vi "De Jitter Data.vi"(10 "Target Info":dbl[][](array[numeric]) format="%#.1f") -> (2 "Filtered Data":dbl[][](array[numeric]))   [LabVIEW 2025]
panel:
  # "Distance"
  # "Angle"
  # "Tag #"
  # "Yaw"
  # "Pitch"
  # "Roll"
  # "Camera #"
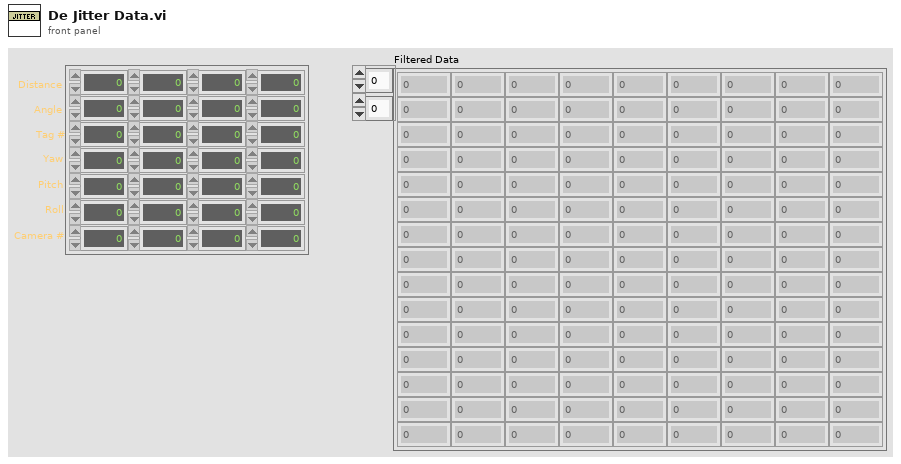
[diagram p1: front panel]
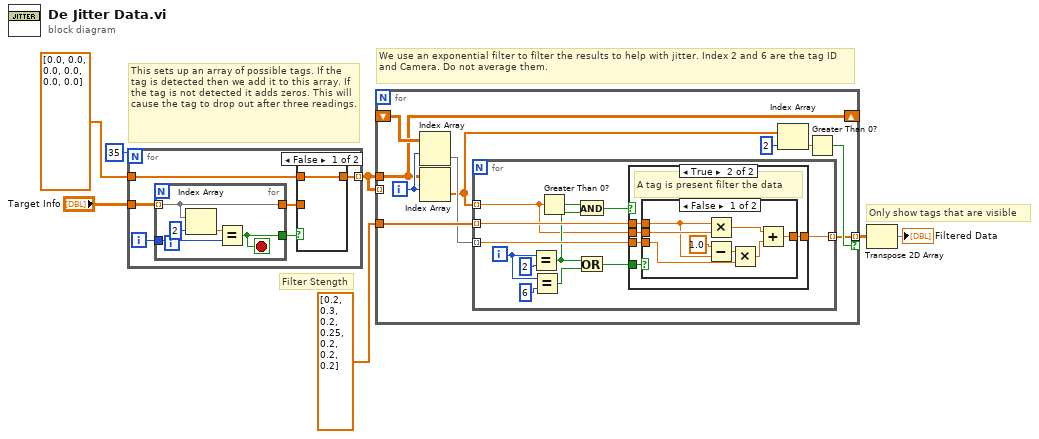
[diagram p0: block diagram]
diagram:
  # "Filter Stength"
  # "Only show tags that are visible"
  # "We use an exponential filter to filter the results to help with jitter. Index 2 and 6 are the tag ID and Camera. Do not average them."
  # "This sets up an array of possible tags. If the tag is detected then we add it to this array. If the tag is not detected it adds zeros. This will cause the tag to drop out after three readings."
  n1 = for {
    N: 35 -> [_]
    tunnel: dbl[] [0.0, 0.0, 0.0, 0.0, 0.0, 0.0] ("f") -> [w10]
    tunnel: "Target Info" -> [w11]
    tunnel: [w9] -> w3 mode=indexing
    i -> [w8]
    n2 = for {
      tunnel: [w15] -> w13
      tunnel: [w16] -> w12
      tunnel: w11 -> [w16] mode=indexing
      tunnel: w8 -> [w17]
      stop <- w15 stop-if-true
      n3 = Index Array(array=w16, index=2) -> (element=w18:dbl)
      n4 = Equal?(x=w18, y=w17) -> (x = y?=w15:bool)
    }
    n5 = case shown="False" w13 {
      tunnel: w12 -> [_ w20]
      tunnel: [w19 w20] -> w9
      tunnel: w10 -> [w19 _]
      frame False {
      }
      frame True {
      }
    }
  }
  n6 = for {
    tunnel: w3 -> [w21]
    shift-right: [w21] -> _
    shift-left: _ -> [w30]
    tunnel: [w28] -> w4 mode=indexing if=w29
    tunnel: w3 -> [_] mode=indexing
    tunnel: dbl[] [0.2, 0.3, 0.2, 0.25, 0.2, 0.2, 0.2] -> [w27]
    i -> [w26]
    n7 = Index Array(array=w30, index (row)=w26) -> (element=w23:dbl[])  [unwired: 1 in]
    n8 = Index Array(array=w21, index (row)=w26) -> (element=w22:dbl[])  [unwired: 1 in]
    n9 = for {
      tunnel: w22 -> [w31] mode=indexing
      tunnel: w23 -> [w42] mode=indexing
      tunnel: [w41] -> w28 mode=indexing
      tunnel: w27 -> [w36] mode=indexing
      i -> [w32]
      n10 = Equal?(x=w32, y=2) -> (x = y?=w34:bool)
      n11 = Equal?(x=w32, y=6) -> (x = y?=w38:bool)
      n12 = Greater Than 0?(x=w31) -> (x > 0?=w33:bool)
      n13 = And(x=w33, y=w34) -> (x .and. y?=w35:bool)
      n14 = Or(x=w34, y=w38) -> (x .or. y?=w37:bool)
      n15 = case shown="True" w35 {
        tunnel: w31 -> [_ w48]
        tunnel: w42 -> [w43 w47]
        tunnel: [w43 w46] -> w41
        tunnel: w37 -> [_ w45]
        tunnel: w36 -> [_ w44]
        frame False {
          # "Tag is 0 Use the previous data"
        }
        frame True {
          # "A tag is present filter the data"
          n16 = case shown="False" w45 {
            tunnel: w48 -> [w56 _]
            tunnel: w47 -> [w53 w57]
            tunnel: [w50 w57] -> w46
            tunnel: w44 -> [w49 _]
            frame False {
              n17 = Multiply(x=w49, y=w56) -> (x*y=w51:dbl)
              n18 = Subtract(x=1.0, y=w49) -> (x-y=w54:dbl)
              n19 = Multiply(x=w54, y=w53) -> (x*y=w52:dbl)
              n20 = Add(x=w51, y=w52) -> (x+y=w50:dbl)
            }
            frame True {
            }
          }
        }
      }
    }
    n21 = Index Array(array=w22, index=2) -> (element=w24:dbl)
    n22 = Greater Than 0?(x=w24) -> (x > 0?=w29:bool)
  }
  n23 = Transpose 2D Array(2D array=w4) -> (transposed array=→"Filtered Data":dbl[][])
